vi "convert % to number(SubVI).vi"(5 "Tolerance":T1) -> (2 "Numeric":dbl)   [LabVIEW 2018]
uses:
  Tolerance.ctl
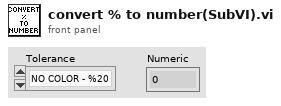
[diagram p1: front panel]
types:
  T1 = typedef "Tolerance.ctl" = enum16{"NO COLOR - %20", "Brown - %1", "Red - %2", "Orange - %3", "Yellow - %4", "Green - %0,5", "Blue - %0,25", "Violet - %0,10", "Grey - %0,05", "Silver x - %10", "Gold x - %5"}
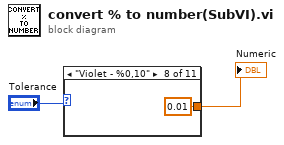
[diagram p0: block diagram]
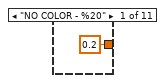
[diagram p2: hidden frame]
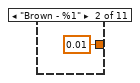
[diagram p3: hidden frame]
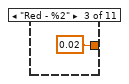
[diagram p4: hidden frame]
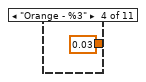
[diagram p5: hidden frame]
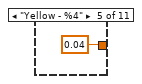
[diagram p6: hidden frame]
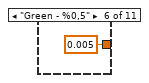
[diagram p7: hidden frame]
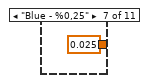
[diagram p8: hidden frame]
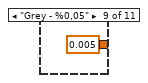
[diagram p9: hidden frame]
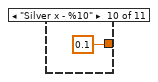
[diagram p10: hidden frame]
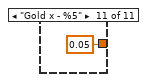
[diagram p11: hidden frame]
diagram:
  n1 = case shown="\"Violet - %0,10\"" "Tolerance" {
    tunnel: [0.2 0.01 0.02 0.03 0.04 0.005 0.025 0.01 0.005 0.1 0.05] -> w1
    frame "NO COLOR - %20" {
    }
    frame "Brown - %1" {
    }
    frame "Red - %2" {
    }
    frame "Orange - %3" {
    }
    frame "Yellow - %4" {
    }
    frame "Green - %0,5" {
    }
    frame "Blue - %0,25" {
    }
    frame "Violet - %0,10" {
    }
    frame "Grey - %0,05" {
    }
    frame "Silver x - %10" {
    }
    frame "Gold x - %5" {
    }
  }
  "Numeric" <- w1
